vi "MCB2300 LED ProjectAttrValidator.vi"(5 "Ctl Refnum":refnum<vi>, 7 "IO Name (original)":string, 9 "LEDNum (0-7)":u32(ring) items=["0", "1", "2", "3", "4", "5", "6", "7"], 11 "Project Attributes":T1 {"Programmable Pin Connections" items=["LED0 and PWM1 use the same pin P2.0. You cannot use LED0 and PWM1 in the same project.", "LED1 and PWM2 use the same pin P2.1. You cannot use LED1 and PWM2 in the same project.", "LED2 and PWM3 use the same pin P2.2. You cannot use LED2 and PWM3 in the same project.", "LED3 and PWM4 use the same pin P2.3. You cannot use LED3 and PWM4 in the same project.", "LED4 and PWM5 use the same pin P2.4. You cannot use LED4 and PWM5 in the same project.", "LED5 and PWM6 use the same pin P2.5. You cannot use LED5 and PWM6 in the same project."]}) -> (3 "Valid?":bool)   [LabVIEW 2011]
uses:
  <vilib>/Embedded/ARM/MCB2300/MCB2300_LED_PrjAttr.ctl
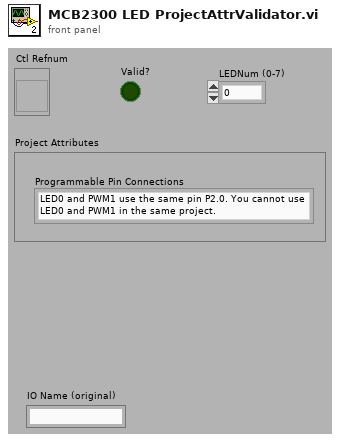
[diagram p1: front panel]
types:
  T1 = typedef "MCB2300_LED_PrjAttr.ctl" = cluster{"Programmable Pin Connections":u16}
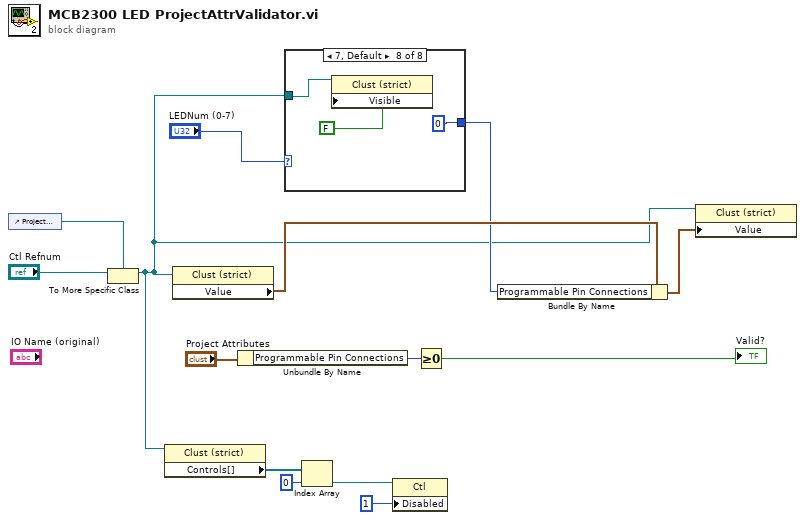
[diagram p0: block diagram]
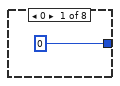
[diagram p2: hidden frame]
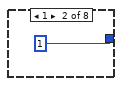
[diagram p3: hidden frame]
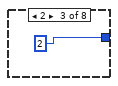
[diagram p4: hidden frame]
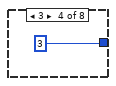
[diagram p5: hidden frame]
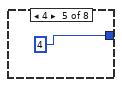
[diagram p6: hidden frame]
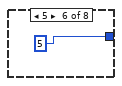
[diagram p7: hidden frame]
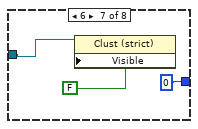
[diagram p8: hidden frame]
diagram:
  n1 = control-ref of="Project Attributes"() -> (w13:refnum<vi>)
  n2 = To More Specific Class(target class=w13, reference="Ctl Refnum") -> (specific class reference=w2:refnum<vi>)  [unwired: 1 in, 1 out]
  n3 = property class="Clust (strict)"(reference=w2) -> ("Controls[]"=w10:refnum<vi>[])  [unwired: 1 in, 2 out]
  n4 = property class="Clust (strict)"(reference=w2) -> ("Value"=w12:cluster{"Programmable Pin Connections":u16})  [unwired: 1 in, 2 out]
  n5 = Unbundle By Name("Project Attributes") -> ("Programmable Pin Connections"=w5:u16)
  n6 = case shown="7, Default" "LEDNum (0-7)" {
    tunnel: [u32 0 u32 1 u32 2 u32 3 u32 4 u32 5 u32 0 u32 0] -> w3
    tunnel: w2 -> [_ _ _ _ _ _ w22 w25]
    frame 0 {
    }
    frame 1 {
    }
    frame 2 {
    }
    frame 3 {
    }
    frame 4 {
    }
    frame 5 {
    }
    frame 6 {
      n7 = property class="Clust (strict)"(reference=w22, "Visible"=FALSE) -> ()  [unwired: 1 in, 2 out]
    }
    frame 7, Default {
      n8 = property class="Clust (strict)"(reference=w25, "Visible"=FALSE) -> ()  [unwired: 1 in, 2 out]
    }
  }
  n9 = Index Array(array=w10, index=0) -> (element=w8:refnum<vi>)
  n10 = property class="Ctl"(reference=w8, "Disabled"=u8 1) -> ()  [unwired: 1 in, 2 out]
  n11 = Greater Or Equal To 0?(x=w5) -> (x >= 0?=→"Valid?":bool)
  n12 = Bundle By Name(cluster=w12, "Programmable Pin Connections"=w3) -> (w11:cluster{"Programmable Pin Connections":u16})
  n13 = property class="Clust (strict)"(reference=w2, "Value"=w11) -> ()  [unwired: 1 in, 2 out]
